vi "Opgave 2.vi"() -> ()   [LabVIEW 2015]
panel:
  out "def F":dbl
  in  "deg C":dbl
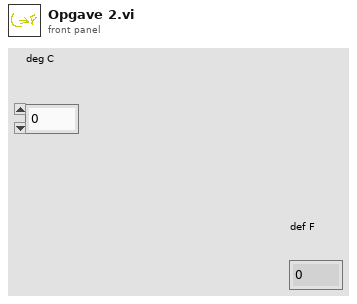
[diagram p1: front panel]
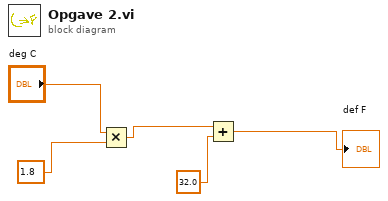
[diagram p0: block diagram]
diagram:
  n1 = Multiply(x="deg C", y=1.8) -> (x*y=w4:dbl)
  n2 = Add(x=w4, y=32.0) -> (x+y=→"def F":dbl)
